vi "create full file path.vi"(8 "error in (no error)":errorcluster, 10 "String":string, 11 "Thorcam in":refnum<class "Thorcam.lvclass">) -> (0 "error out":errorcluster, 2 "full file path":path, 3 "Thorcam out":refnum<class "Thorcam.lvclass">)   [LabVIEW 2012, in "Thorcam.lvclass"]
uses:
  Thorcam.lvclass
  Thorcam.lvclass/Thorcam.ctl
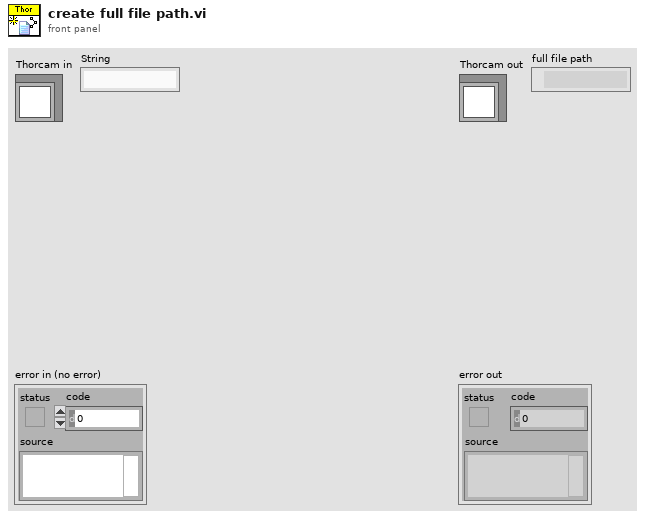
[diagram p1: front panel]
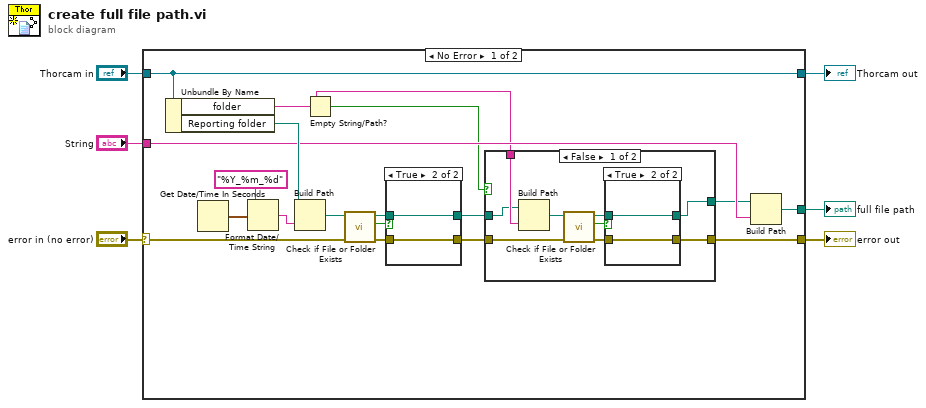
[diagram p0: block diagram]
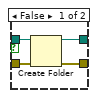
[diagram p2: hidden frame]
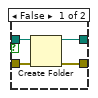
[diagram p4: hidden frame]
diagram:
  n1 = case shown="No Error" "error in (no error)" {
    selector: "error in (no error)" -> [w18 w49]
    tunnel: [w10 w49] -> w5
    tunnel: [w24 w48] -> w3
    tunnel: "Thorcam in" -> [w24 w48]
    tunnel: "String" -> [w13 _]
    tunnel: [w14 _] -> w1
    frame No Error {
      n2 = Unbundle By Name(w24) -> ("folder"=w7:string, "Reporting folder"=w20:path)
      n3 = Get Date/Time In Seconds() -> (seconds since 1Jan1904=w23:timestamp)
      n4 = Format Date/Time String(time format string (%c)="%Y_%m_%d", seconds (now)=w23) -> (date/time string=w21:string)  [unwired: 1 in]
      n5 = Build Path(base path=w20, name or relative path=w21) -> (appended path=w19:path)
      n6 = Empty String/Path?(string/path=w7) -> (empty?=w12:bool)
      n7 = call <vilib>:"Check if File or Folder Exists.vi"("error in (no error)"=w18, "path"=w19) -> ("error out"=w16:errorcluster, "file or folder exists?"=w17:bool, "dup path"=w15:path)  [unwired: 7 in]
      n8 = case shown="True" w17 {
        tunnel: w16 -> [w45 w47]
        tunnel: w15 -> [w44 w46]
        tunnel: [w43 w47] -> w9
        tunnel: [w42 w46] -> w11
        frame False {
          n9 = Create Folder(path (use dialog)=w44, error in=w45) -> (created path=w42:path, error out=w43:errorcluster)  [unwired: 1 in, 1 out]
        }
        frame True {
        }
      }
      n10 = case shown="False" w12 {
        tunnel: w11 -> [w27 w40]
        tunnel: [w25 w41] -> w10
        tunnel: w9 -> [w29 w41]
        tunnel: [w26 w40] -> w8
        tunnel: w7 -> [w28 _]
        frame False {
          n11 = Build Path(base path=w27, name or relative path=w28) -> (appended path=w33:path)
          n12 = call <vilib>:"Check if File or Folder Exists.vi"("error in (no error)"=w29, "path"=w33) -> ("error out"=w31:errorcluster, "file or folder exists?"=w32:bool, "dup path"=w30:path)  [unwired: 7 in]
          n13 = case shown="True" w32 {
            tunnel: w31 -> [w37 w39]
            tunnel: w30 -> [w36 w38]
            tunnel: [w35 w39] -> w25
            tunnel: [w34 w38] -> w26
            frame False {
              n14 = Create Folder(path (use dialog)=w36, error in=w37) -> (created path=w34:path, error out=w35:errorcluster)  [unwired: 1 in, 1 out]
            }
            frame True {
            }
          }
        }
        frame True {
        }
      }
      n15 = Build Path(base path=w8, name or relative path=w13) -> (appended path=w14:path)
    }
    frame Error {
    }
  }
  "error out" <- w5
  "Thorcam out" <- w3
  "full file path" <- w1
